vi "Send path to matlab.vi"(8 "error in":errorcluster) -> (0 "error out":errorcluster)   [LabVIEW 2020]
uses:
  Global Variables/General Globals.vi
panel:
  out "Execution time (ms)":u32
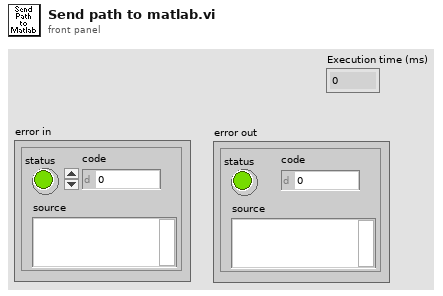
[diagram p1: front panel]
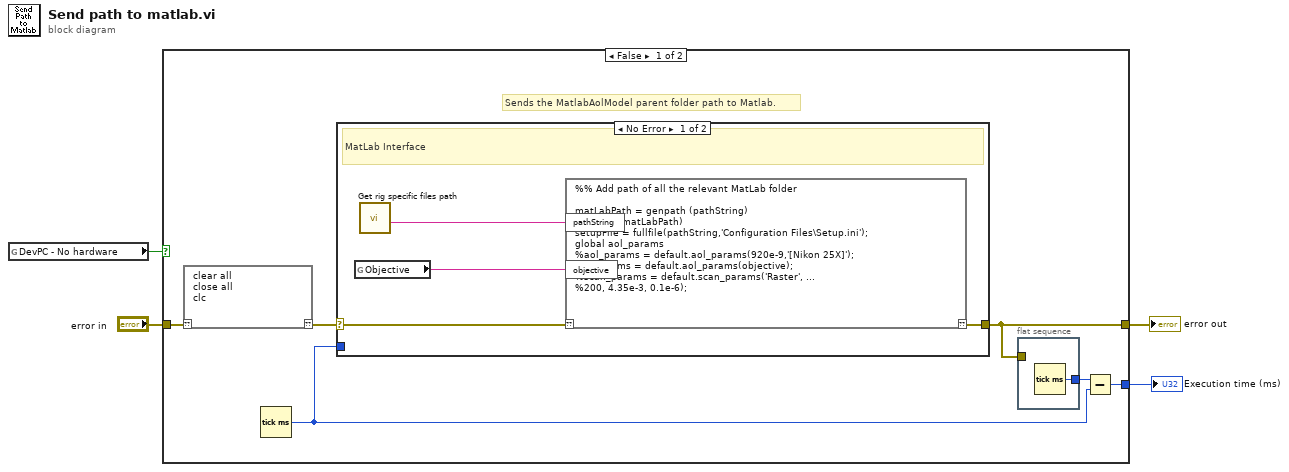
[diagram p0: block diagram]
diagram:
  n1 = global read "General Globals.vi" "DevPC - No hardware"() -> (w1:bool)
  n2 = case shown="False" w1 {
    tunnel: "error in" -> [w10 w17]
    tunnel: [w6 _] -> w3
    tunnel: [w5 w17] -> w2
    frame False {
      # "Sends the MatlabAolModel parent folder path to Matlab."
      n3 = script code="clear all\nclose all\nclc"("??"=w10) -> ("??"=w9:errorcluster)
      n4 = Tick Count (ms)() -> (millisecond timer value=w7:u32)
      n5 = case shown="No Error" w9 {
        selector: w9 -> [w15 w16]
        tunnel: [w14 w16] -> w5
        tunnel: w7 -> [_ _]
        frame No Error {
          # "MatLab Interface"
          n6 = global read "General Globals.vi" "Objective"() -> (w12:string)
          n7 = call "Get rig specific files path.vi"() -> ("Rig-specific files folder (string)"=w13:string)  [unwired: 10 in, 1 out]
          n8 = script code="%% Add path of all the relevant MatLab folder\n\nmatLabPath = genpath (pathString)\naddpath (matLabPath)\nsetupFile = fullfile(pathString,'Configuration Files\\Setup.ini');\nglobal aol_params\n%aol_params = default.aol_params(920e-9,'[Nikon 25X]');\naol_params = default.aol_params(objective);\n%scan_params = default.scan_params('Raster', ...\n%200, 4.35e-3, 0.1e-6);"("??"=w15, "pathString"=w13, "objective"=w12) -> ("??"=w14:errorcluster)
        }
        frame Error {
        }
      }
      n9 = flat-sequence {
        tunnel: [w11] -> w8
        tunnel: w5 -> [_]
        frame #0 {
          n10 = Tick Count (ms)() -> (millisecond timer value=w11:u32)
        }
      }
      n11 = Subtract(x=w8, y=w7) -> (x-y=w6:u32)
    }
    frame True {
      # "Demo mode / No hardware"
    }
  }
  "error out" <- w2
  "Execution time (ms)" <- w3
